vi "Finger_Position_Compute.vi"(9 "Max Distance":dbl[](array[numeric]), 10 "Hand Position":cluster{"X":dbl, "Y":dbl, "Z":dbl}, 11 "Finger Positions":T1(array[cluster])) -> (1 "Max Distance out":dbl[](array[numeric]), 2 "Finger position":dbl[](array[numeric]))   [LabVIEW 2015]
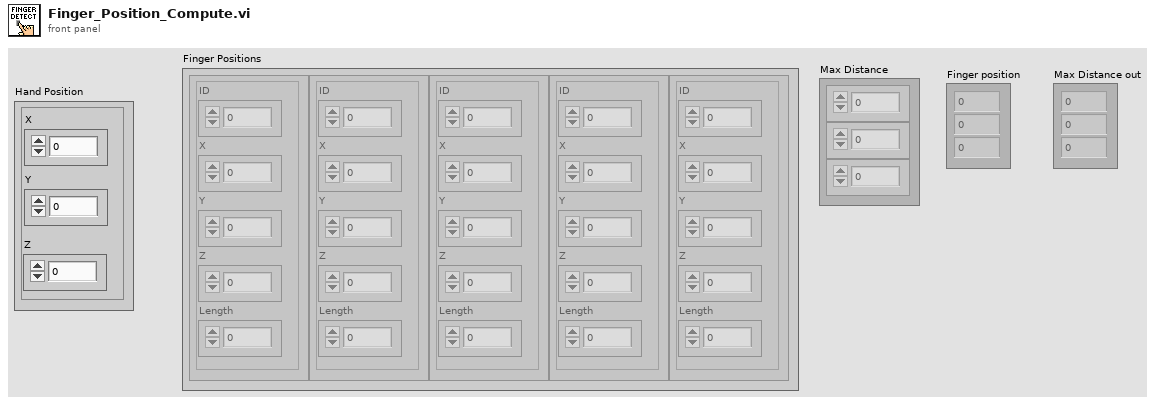
[diagram p1: front panel]
types:
  T1 = cluster{"ID":dbl, "X":dbl, "Y":dbl, "Z":dbl, "Length":dbl}[]
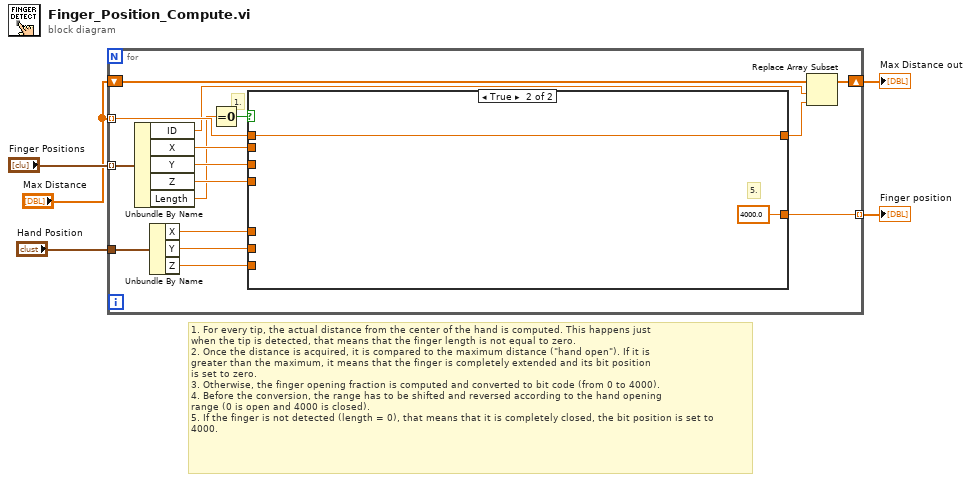
[diagram p0: block diagram]
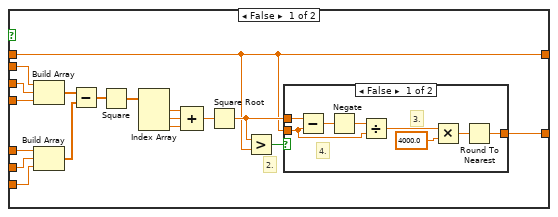
[diagram p2: hidden frame]
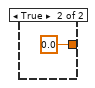
[diagram p3: hidden frame]
diagram:
  # "1. For every tip, the actual distance from the center of the hand is computed. This happens just\nwhen the tip is detected, that means that the finger length is not equal to zero.\n2. Once the distance is acquired, it is compared to the maximum distance (\"hand open\"). If it is \ngreater than the maximum, it means that the finger is completely extended and its bit position \nis set to zero.\n3. Otherwise, the finger opening fraction is computed and converted to bit code (from 0 to 4000).\n4. Before the conversion, the range has to be shifted and reversed according to the hand opening\nrange (0 is open and 4000 is closed).\n5. If the finger is not detected (length = 0), that means that it is completely closed, the bit position is set to \n4000."
  n1 = for {
    tunnel: "Hand Position" -> [w12]
    tunnel: "Finger Positions" -> [w21] mode=indexing
    tunnel: [w14] -> w3 mode=indexing
    tunnel: "Max Distance" -> [w13] mode=indexing
    shift-right: [w11] -> w2
    shift-left: "Max Distance" -> [w10]
    # "1."
    n2 = Unbundle By Name(w21) -> ("ID"=w8:dbl, "X"=w20:dbl, "Y"=w19:dbl, "Z"=w18:dbl, "Length"=w6:dbl)
    n3 = Unbundle By Name(w12) -> ("X"=w17:dbl, "Y"=w16:dbl, "Z"=w15:dbl)
    n4 = Equal To 0?(x=w6) -> (x = 0?=w7:bool)
    n5 = case shown="True" w7 {
      tunnel: w20 -> [w37 _]
      tunnel: w19 -> [w36 _]
      tunnel: w18 -> [w35 _]
      tunnel: w17 -> [w34 _]
      tunnel: w16 -> [w33 _]
      tunnel: w15 -> [w32 _]
      tunnel: [w25 sgl 4000.0 ("y")] -> w14
      tunnel: w13 -> [w23 w49]
      tunnel: [w23 w49] -> w9
      frame False {
        # "2."
        n6 = Build Array(w37, w36, w35) -> (w30:dbl[])
        n7 = Build Array(w34, w33, w32) -> (w31:dbl[])
        n8 = Subtract(x=w30, y=w31) -> (x-y=w39:dbl[])
        n9 = Square(x=w39) -> (x^2=w29:dbl[])
        n10 = Index Array(array=w29) -> (element #1=w28:dbl, element #2=w27:dbl, element #3=w26:dbl)  [unwired: 3 in]
        n11 = Compound Arithmetic op=ADD(w28, w27, w26) -> (w38:dbl)
        n12 = Square Root(x=w38) -> (sqrt(x)=w24:dbl)
        n13 = Greater?(x=w24, y=w23) -> (0:w22:bool)
        n14 = case shown="False" w22 {
          tunnel: [w45 0.0] -> w25
          tunnel: w24 -> [w41 _]
          tunnel: w23 -> [w40 _]
          frame False {
            # "4."
            # "3."
            n15 = Subtract(x=w41, y=w40) -> (x-y=w44:dbl)
            n16 = Negate(x=w44) -> (-x=w43:dbl)
            n17 = Divide(x=w43, y=w40) -> (x/y=w46:dbl)
            n18 = Multiply(x=w46, y=sgl 4000.0) -> (x*y=w47:dbl)
            n19 = Round To Nearest(number=w47) -> (nearest integer value=w45:dbl)
          }
          frame True {
          }
        }
      }
      frame True {
        # "5."
      }
    }
    n20 = Replace Array Subset(array=w10, new element=w9, index=w8) -> (w11:dbl[])
  }
  "Finger position" <- w3
  "Max Distance out" <- w2
